vi "DefendGoalTacticVSS.vi"(7 "First call?":bool=TRUE, 9 "Game in":refnum<class "Game.lvclass">, 10 "Robot":refnum<class "Robot.lvclass">, 11 "DefendGoalTacticVSS in":refnum<class "DefendGoalTacticVSS.lvclass">) -> (2 "Robot out":refnum<class "Robot.lvclass">, 3 "DefendGoalTacticVSS out":refnum<class "DefendGoalTacticVSS.lvclass">)   [LabVIEW 2023, in "DefendGoalTacticVSS.lvclass"]
uses:
  DefendGoalTacticVSS.lvclass
  Robot_class/Robot.lvclass
  Game_class/Game.lvclass
  C:/Users/roboi/Downloads/VSS_AI-Larc2023 - Copia (2)/Tactic_class/Tactic.lvclass
  Robot_class/tactics.ctl
  DefendGoalStates.ctl
  Tactic_class/Tactic.lvclass/Tactic.ctl
  Game_class/Game.lvclass/Game.ctl
  DefendGoalTacticVSS.lvclass/DefendGoalTacticVSS.ctl
  Robot_class/Robot.lvclass/Robot.ctl
  Game_class/Read BallRef.vi
  Tactic_class/Read Skillbook.vi
  Robot_class/Write tactic.vi
  Write States.vi
  Skillbook_class/Skillbook.lvclass
  Ball_class/Ball.lvclass
  KickSkillVSS_class/KickSkillVSS.lvclass
  PenaltyPosSkillVSS_class/PenaltyPosSkillVSS.lvclass
  BallDispPosSkillVSS_class/BallDispPosSkillVSS.lvclass
  BallToGoalSkillVSS_class/BallToGoalSkillVSS.lvclass
  GoToBallSkillVSS_class/GoToBallSkillVSS.lvclass
  DefBallPosSkillVSS_class/DefBallPosSkillVSS.lvclass
  HaltSkill_class/HaltSkill.lvclass
  KeeperDefPosSkillVSS_class/KeeperDefPosSkillVSS.lvclass
  GoToBallKeeperSkillVSS_class/GoToBallKeeperSkillVSS.lvclass
  RotateWallSkillVSS_class/RotateWallSkillVSS.lvclass
panel:
  out "x .or. y?":bool
  out "error out 2":errorcluster
  in  "error in (no error) 2":errorcluster
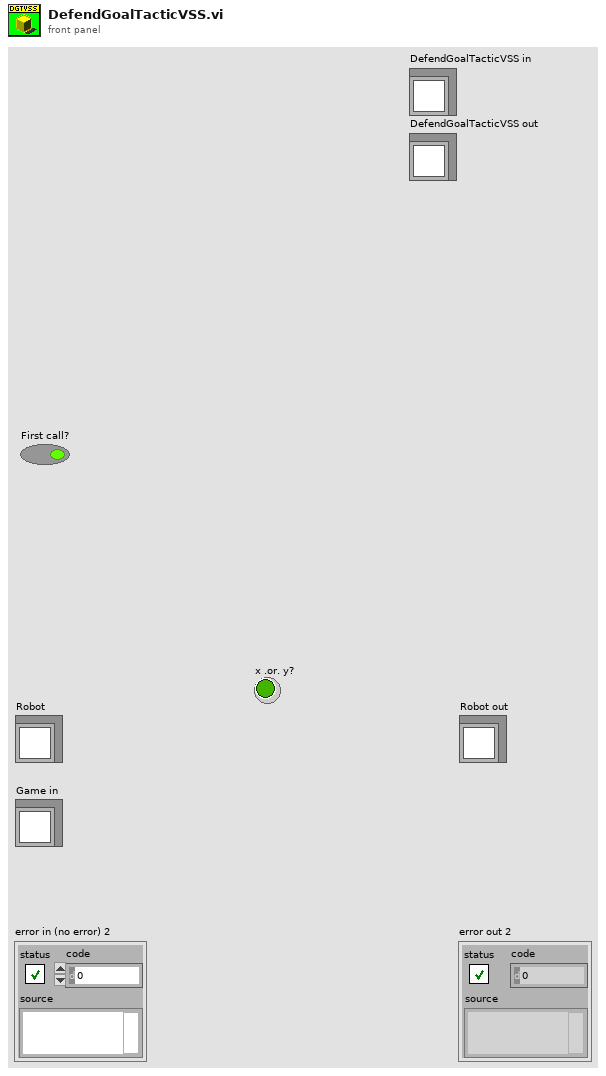
[diagram p1: front panel]
types:
  T1 = typedef "DefendGoalStates.ctl" = enum16{"Kick", "DefBallPos", "SpillSkin", "Exit"}
  T2 = typedef "tactics.ctl" = enum16{"ReceivePassInFuturePoint", "Roller", "PrepareRollToPassRollerGoTo", "PrepareRollToPassReceiverGoTo", "WaitRoll", "PositionToRoll", "PenaltyAttacker", "PassObserver", "PenaltyDefense", "TableReceiverTactic", "Test", "DefendGoal", "Marker", "FollowAttacker", "DefendArea", "Shoot", "AttackerAimGoal", "AttackerBallOutOfField", "AttackerBlock", "AttackerStop", "Duelist", "Halt", "ZigZag", "GoTo", "Timeout", "KickToPassReceiver", "PositionToReceivePass", "DefendAreaVSS", "DefendGoalVSS", "KickVSS", "AttackVSS", "DispBallVSS", "PenaltyAttackVSS", "WaitPass"}
  T3 = cluster{"KickSkillVSS":refnum<class "KickSkillVSS.lvclass">, "PenaltyPosSkillVSS":refnum<class "PenaltyPosSkillVSS.lvclass">, "BallDispPosSkillVSS":refnum<class "BallDispPosSkillVSS.lvclass">, "BallToGoalSkillVSS":refnum<class "BallToGoalSkillVSS.lvclass">, "GoToBallSkillVSS":refnum<class "GoToBallSkillVSS.lvclass">, "DefBallPosSkillVSS":refnum<class "DefBallPosSkillVSS.lvclass">, "HaltSkill":refnum<class "HaltSkill.lvclass">, "KeeperDefPosSkillVSS":refnum<class "KeeperDefPosSkillVSS.lvclass">, "GoToBallKeeperSkillVSS":refnum<class "GoToBallKeeperSkillVSS.lvclass">, "RotateWallSkillVSS":refnum<class "RotateWallSkillVSS.lvclass">}
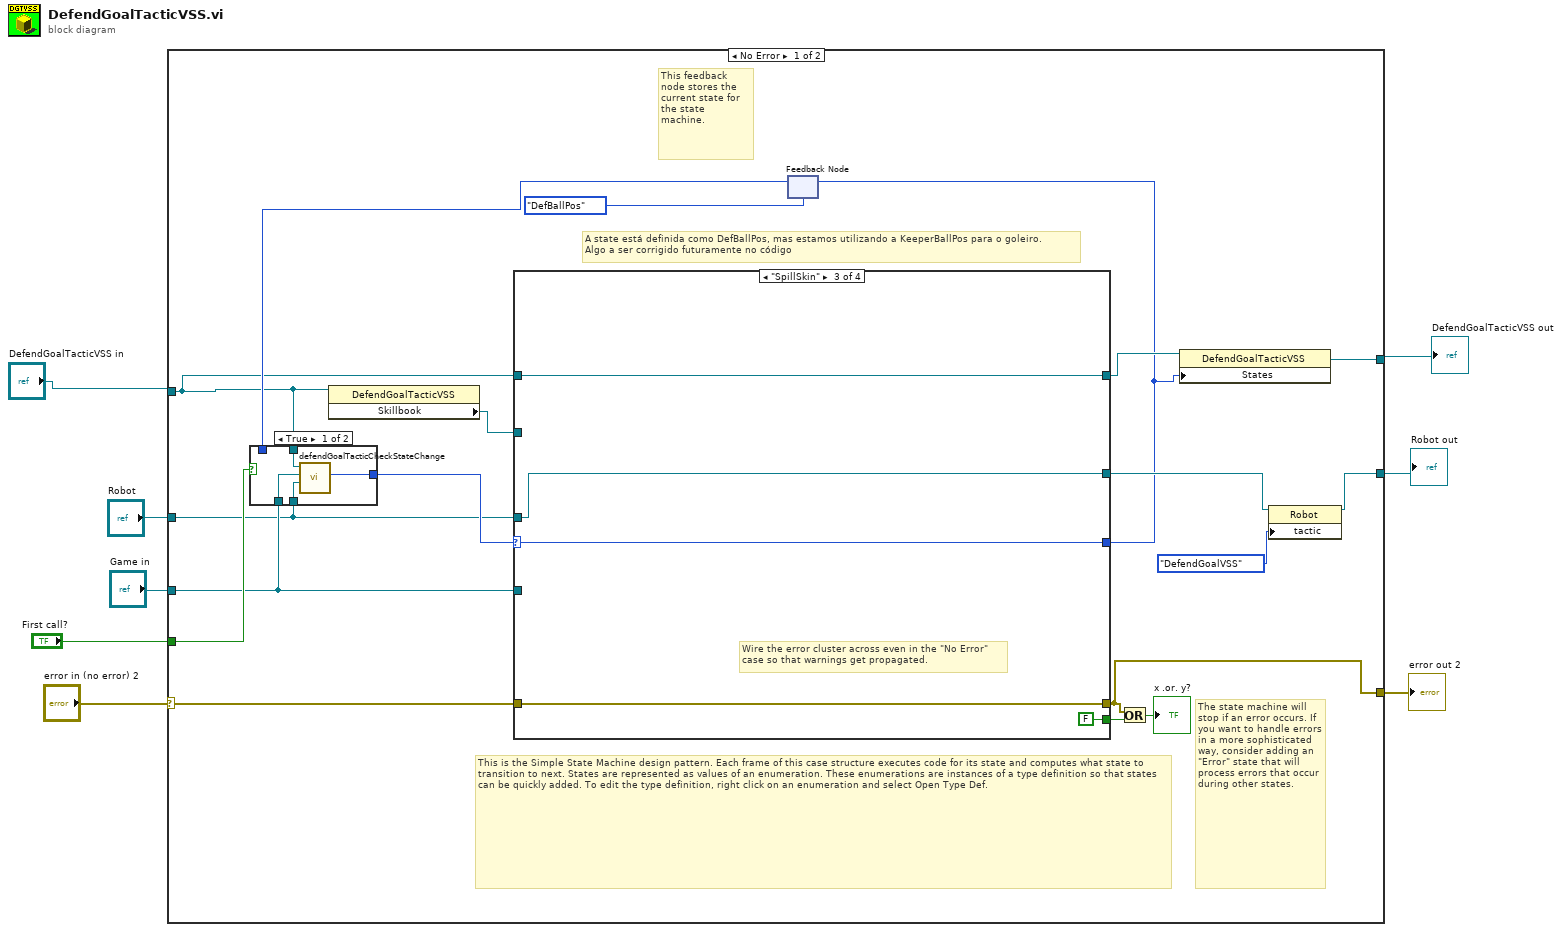
[diagram p0: block diagram]
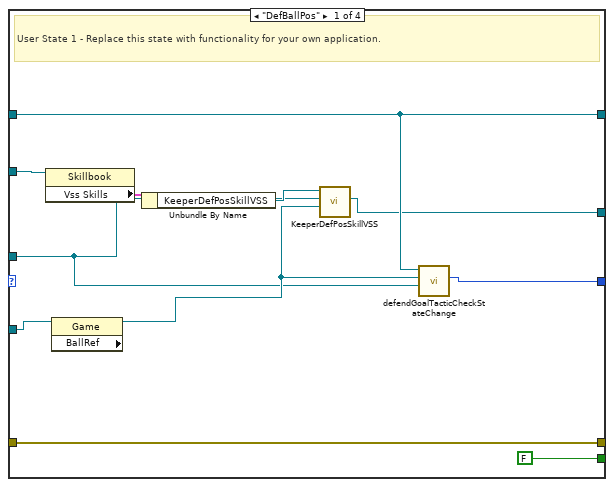
[diagram p3: hidden frame]
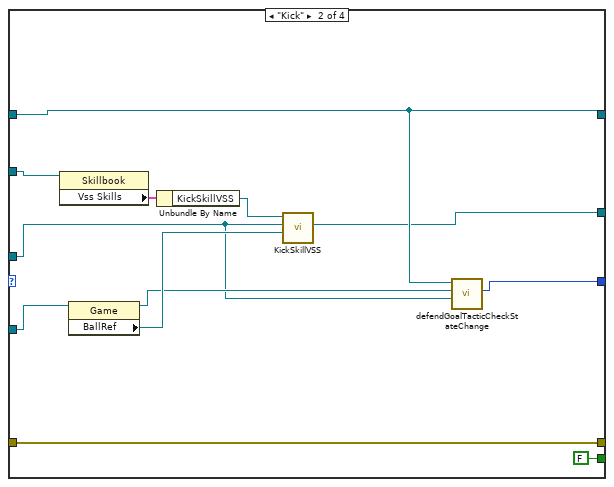
[diagram p4: hidden frame]
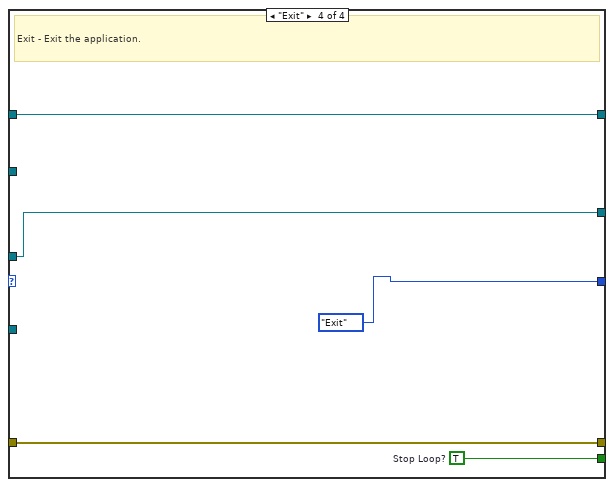
[diagram p5: hidden frame]
diagram:
  n1 = case shown="No Error" "error in (no error) 2" {
    selector: "error in (no error) 2" -> [w22 w67]
    tunnel: [w21 w67] -> w7
    tunnel: [w20 w66] -> w2
    tunnel: "DefendGoalTacticVSS in" -> [w10 w66]
    tunnel: "Robot" -> [w11 w65]
    tunnel: "Game in" -> [w14 _]
    tunnel: [w17 w65] -> w4
    tunnel: "First call?" -> [w15 _]
    frame No Error {
      # "A state está definida como DefBallPos, mas estamos utilizando a KeeperBallPos para o goleiro.\nAlgo a ser corrigido futuramente no código"
      # "The state machine will stop if an error occurs. If you want to handle errors in a more sophisticated way, consider adding an \"Error\" state that will process errors that occur during other states."
      # "This feedback node stores the current state for the state machine."
      # "This is the Simple State Machine design pattern. Each frame of this case structure executes code for its state and computes what state to transition to next. States are represented as values of an enumeration. These enumerations are instances of a type definition so that states can be quickly added. To edit the type definition, right click on an enumeration and select Open Type Def."
      # "Wire the error cluster across even in the \"No Error\"\ncase so that warnings get propagated."
      n2 = property class="DefendGoalTacticVSS"(reference=w10) -> ("Skillbook"=w24:refnum<class "Skillbook.lvclass">)  [unwired: 1 in, 2 out]
      n3 = feedback #1(DefendGoalStates."DefBallPos" ("States")) -> (w13:T1)
      n4 = case shown="True" w15 {
        tunnel: w10 -> [w30 _]
        tunnel: w11 -> [w29 _]
        tunnel: w14 -> [w28 _]
        tunnel: [w27 w31] -> w12
        tunnel: w13 -> [_ w31]
        frame True {
          n5 = call "defendGoalTacticCheckStateChange.vi"("Robot In"=w29, "Game in"=w28, "DefendGoalTacticVSS in"=w30) -> ("States"=w27:T1)  [unwired: 6 in, 2 out]
        }
        frame False {
        }
      }
      n6 = case shown="\"SpillSkin\"" w12 {
        selector: w12 -> [_ _ w56 _]
        tunnel: [w38 w53 w56 DefendGoalStates."Exit" ("States")] -> w9
        tunnel: [FALSE ("Stop Loop?") FALSE ("Stop Loop?") FALSE ("Stop Loop?") w64] -> w26
        tunnel: w24 -> [w41 w51 _ _]
        tunnel: w11 -> [w32 w43 w58 w63]
        tunnel: [w33 w52 w58 w63] -> w18
        tunnel: [w37 w54 w59 w62] -> w23
        tunnel: w10 -> [w37 w54 w59 w62]
        tunnel: w14 -> [w36 w46 _ _]
        tunnel: [w40 w48 w57 w61] -> w21
        tunnel: w22 -> [w40 w48 w57 w61]
        frame "DefBallPos" {
          # "User State 1 - Replace this state with functionality for your own application."
          n7 = property class="Skillbook"(reference=w41) -> ("Vss Skills"=w39:T3)  [unwired: 1 in, 2 out]
          n8 = property class="Game" props=["BallRef"](reference=w36) -> (reference out=w34:refnum<class "Game.lvclass">)  [unwired: 1 in, 2 out]
          n9 = Unbundle By Name(w39) -> ("KeeperDefPosSkillVSS"=w35:refnum<class "KeeperDefPosSkillVSS.lvclass">)
          n10 = call "KeeperDefPosSkillVSS.vi"("Game"=w34, "Robot in"=w32, "KeeperDefPosSkillVSS in"=w35) -> ("Robot out"=w33:refnum<class "Robot.lvclass">)  [unwired: 6 in, 2 out]
          n11 = call "defendGoalTacticCheckStateChange.vi"("Robot In"=w32, "Game in"=w34, "DefendGoalTacticVSS in"=w37) -> ("States"=w38:T1)  [unwired: 6 in, 2 out]
        }
        frame "Kick" {
          n12 = property class="Skillbook"(reference=w51) -> ("Vss Skills"=w50:T3)  [unwired: 1 in, 2 out]
          n13 = property class="Game"(reference=w46) -> (reference out=w44:refnum<class "Game.lvclass">, "BallRef"=w45:refnum<class "Ball.lvclass">)  [unwired: 1 in, 1 out]
          n14 = Unbundle By Name(w50) -> ("KickSkillVSS"=w49:refnum<class "KickSkillVSS.lvclass">)
          n15 = call-dynamic "KickSkillVSS.vi"("BallRef"=w45, "Robot"=w43, "KickSkillVSS in"=w49) -> ("Robot out"=w52:refnum<class "Robot.lvclass">)  [unwired: 6 in, 2 out]
          n16 = call "defendGoalTacticCheckStateChange.vi"("Robot In"=w43, "Game in"=w44, "DefendGoalTacticVSS in"=w54) -> ("States"=w53:T1)  [unwired: 6 in, 2 out]
        }
        frame "SpillSkin" {
        }
        frame "Exit" {
          w64 = TRUE  # Stop Loop?
          # "Exit - Exit the application."
        }
      }
      n17 = feedback-in #1(w9) -> ()
      n18 = Or(x=w21, y=w26) -> (x .or. y?=→"x .or. y?":bool)
      n19 = property class="DefendGoalTacticVSS"(reference=w23, "States"=w9) -> (reference out=w20:refnum<class "DefendGoalTacticVSS.lvclass">)  [unwired: 1 in, 1 out]
      n20 = property class="Robot"(reference=w18, "tactic"=tactics."DefendGoalVSS") -> (reference out=w17:refnum<class "Robot.lvclass">)  [unwired: 1 in, 1 out]
    }
    frame Error {
    }
  }
  "error out 2" <- w7
  "Robot out" <- w4
  "DefendGoalTacticVSS out" <- w2
